vi "Clean.vi"(10 "Split Key":string, 11 "Filenames In":string[](array[string])) -> (3 "Filenames Out":string[](array[string]))   [LabVIEW 2024]
uses:
  <vilib>/Utility/error.llb/whitespace.ctl
  <vilib>/Utility/error.llb/Trim Whitespace One-Sided.vi
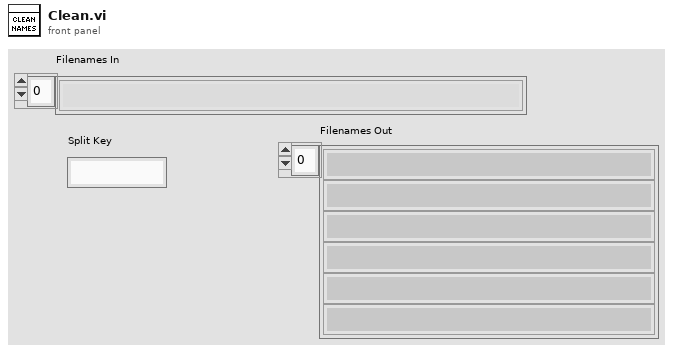
[diagram p1: front panel]
types:
  T1 = typedef "whitespace.ctl" = u16
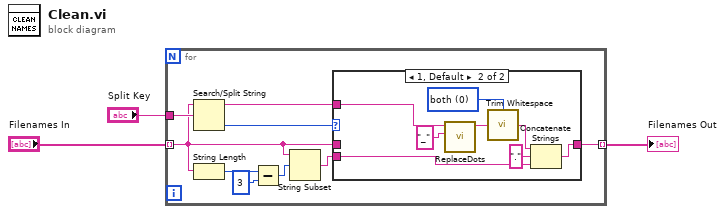
[diagram p0: block diagram]
diagram:
  n1 = for {
    tunnel: "Filenames In" -> [w5] mode=indexing
    tunnel: "Split Key" -> [w11]
    tunnel: [w9] -> w2 mode=indexing
    n2 = Search/Split String(string=w5, search string/char (-)=w11) -> (substring before match=w12:string, offset of match=w10:i32)  [unwired: 1 in, 1 out]
    n3 = String Length(string=w5) -> (length=w8:i32)
    n4 = Subtract(x=w8, y=3) -> (x-y=w4:i32)
    n5 = String Subset(string=w5, offset (0)=w4) -> (substring=w6:string)  [unwired: 1 in]
    n6 = case shown="1, Default" w10 {
      tunnel: w12 -> [_ w14]
      tunnel: w6 -> [_ w16]
      tunnel: [w13 w21] -> w9
      tunnel: w5 -> [w13 _]
      frame -1 {
      }
      frame 1, Default {
        w17 = T1 0 items=["both", "start of string", "end of string"] ("location (both)")
        n7 = call "ReplaceDots.vi"("search string"="_", "String In"=w14) -> ("String Out"=w19:string)  [unwired: 8 in, 1 out]
        n8 = call <vilib>:"Trim Whitespace.vi"("string"=w19, "location (both)"=w17) -> ("trimmed string"=w18:string)
        n9 = Concatenate Strings(w18, "." ("string"), w16) -> (w21:string)
      }
    }
  }
  "Filenames Out" <- w2
